vi "LV2GCRCLookup.vi"(7 "Operation":T1, 8 "error in (no error)":errorcluster, 11 "Lookup":string[][](array[string])) -> (0 "error out":errorcluster, 3 "Lookup Out":string[][](array[string]))   [LabVIEW 2018]
uses:
  <vilib>/Utility/file.llb/Write To Spreadsheet File (string).vi
  <vilib>/Utility/file.llb/Read From Spreadsheet File (string).vi
  Strict Type Controls/Settings Operation.ctl
panel:
  # "N1\t93,81\nN2\t157,81\nN3\t92,114\nN4\t157,80"
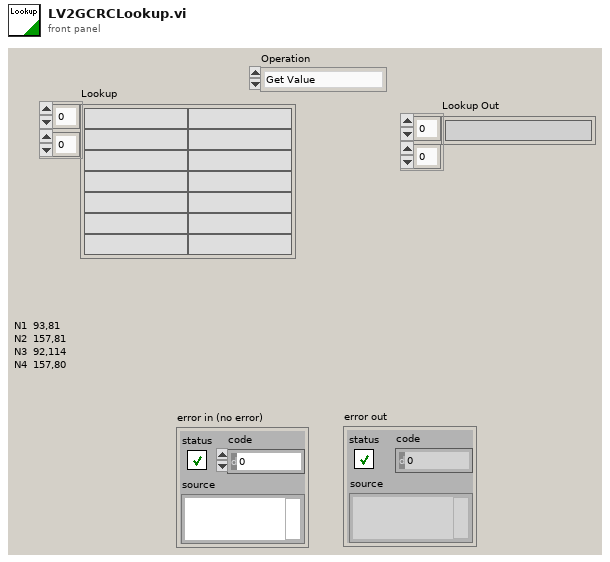
[diagram p1: front panel]
types:
  T1 = typedef "Settings Operation.ctl" = enum8{"Get Value", "Set Value", "Read File", "Write File", "Write Stored Value"}
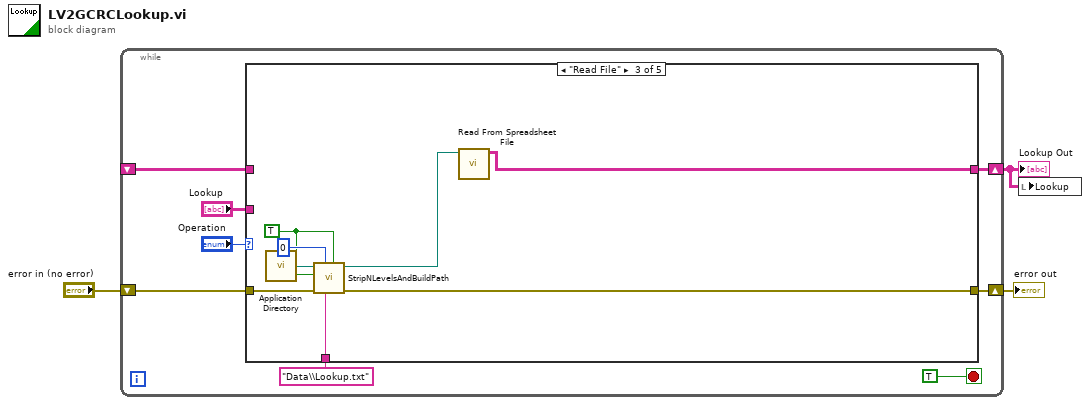
[diagram p0: block diagram]
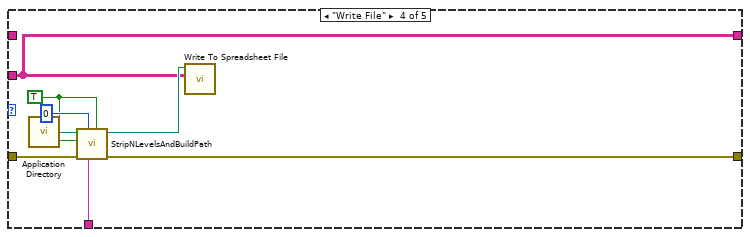
[diagram p4: hidden frame]
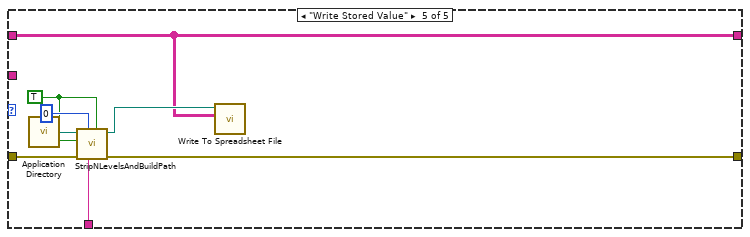
[diagram p5: hidden frame]
diagram:
  n1 = while {
    shift-right: [w10] -> w1
    shift-left: _ -> [w11]
    shift-right: [w7] -> w2
    shift-left: "error in (no error)" -> [w8]
    stop <- TRUE stop-if-true
    n2 = case shown="\"Read File\"" "Operation" {
      tunnel: w11 -> [w13 _ _ _ w33]
      tunnel: [w13 w15 w17 w25 w33] -> w10
      tunnel: "Lookup" -> [_ w15 _ w25 _]
      tunnel: w8 -> [w12 w14 w20 w30 w36]
      tunnel: [w12 w14 w16 w24 w32] -> w7
      tunnel: "Data\\Lookup.txt" ("Build Path") -> [_ _ w19 w27 w35]
      frame "Get Value" {
      }
      frame "Set Value" {
      }
      frame "Read File" {
        w21 = TRUE ("Is File?")
        n3 = call <vilib>:"Application Directory.vi"() -> ("Application Directory"=w23:path)
        n4 = call "StripNLevelsAndBuildPath.vi"("Create Folders"=w21, "Build Path"=w19, "Strip Levels"=0, "error in(no error)"=w20, "Is File"=w21, "Path In"=w23) -> ("error out"=w16:errorcluster, "Path Out"=w18:path)  [unwired: 4 out]
        n5 = call-poly <vilib>:"Read From Spreadsheet File.vi"("file path (dialog if empty)"=w18) -> ("all rows"=w17:string[][])  [unwired: 6 in, 4 out]
      }
      frame "Write File" {
        w28 = TRUE ("Is File?")
        n6 = call <vilib>:"Application Directory.vi"() -> ("Application Directory"=w31:path)
        n7 = call "StripNLevelsAndBuildPath.vi"("Create Folders"=w28, "Build Path"=w27, "Strip Levels"=0, "error in(no error)"=w30, "Is File"=w28, "Path In"=w31) -> ("error out"=w24:errorcluster, "Path Out"=w26:path)  [unwired: 4 out]
        n8 = call-poly <vilib>:"Write To Spreadsheet File.vi"("2D data"=w25, "file path (dialog if empty)"=w26) -> ()  [unwired: 6 in, 1 out]
      }
      frame "Write Stored Value" {
        w37 = TRUE ("Is File?")
        n9 = call <vilib>:"Application Directory.vi"() -> ("Application Directory"=w39:path)
        n10 = call "StripNLevelsAndBuildPath.vi"("Create Folders"=w37, "Build Path"=w35, "Strip Levels"=0, "error in(no error)"=w36, "Is File"=w37, "Path In"=w39) -> ("error out"=w32:errorcluster, "Path Out"=w34:path)  [unwired: 4 out]
        n11 = call-poly <vilib>:"Write To Spreadsheet File.vi"("2D data"=w33, "file path (dialog if empty)"=w34) -> ()  [unwired: 6 in, 1 out]
      }
    }
  }
  "error out" <- w2
  "Lookup Out" <- w1
  n12 = local write "Lookup"(w1) -> ()
